vi "Dir_Pad_To_Value_Debug.vi"() -> ()   [LabVIEW 2011]
panel:
  out "Pos_Pad_Val":i32
  in  "Axis_6_Val":dbl
  in  "Axis_5_Val":dbl
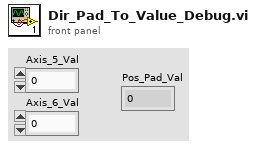
[diagram p1: front panel]
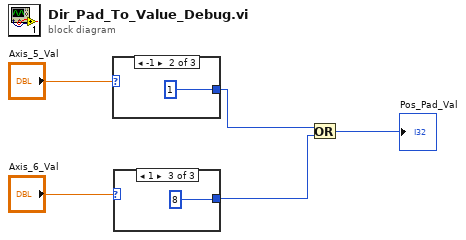
[diagram p0: block diagram]
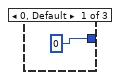
[diagram p2: hidden frame]
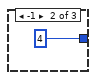
[diagram p3: hidden frame]
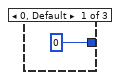
[diagram p4: hidden frame]
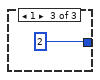
[diagram p5: hidden frame]
diagram:
  n1 = case shown="-1" "Axis_5_Val" {
    tunnel: [0 1 2] -> w3
    frame 0, Default {
    }
    frame -1 {
    }
    frame 1 {
    }
  }
  n2 = case shown="1" "Axis_6_Val" {
    tunnel: [0 4 8] -> w2
    frame 0, Default {
    }
    frame -1 {
    }
    frame 1 {
    }
  }
  n3 = Or(x=w3, y=w2) -> (x .or. y?=→"Pos_Pad_Val":i32)
